vi "Acquisition-ACQUIRE case.vi"(1 "Message Queues":T1, 5 "Logging queue in":T3, 9 "Acquired z-plane index":i32) -> (4 "Imaging Protocol":T2=enum."Live Imaging", 6 "VI Exec time":u32, 10 "Index of next Z-plane to acquire":i32, 15 "Error Out":errorcluster)   [LabVIEW 2020]
doc: "Perform the acquisition. Replace the contents of this diagram with calls to acquisition hardware."
uses:
  Typedefs/Data queue ref.ctl
  Typedefs/Logging queue element.ctl
  Typedefs/Imaging Protocols enum.ctl
  Typedefs/Frame Size.ctl
  Typedefs/Acquired points count.ctl
  User Interface/Queue/Message Queue/Typedefs/All Message Queues.ctl
  User Interface/Queue/Message Queue/Typedefs/Message Cluster.ctl
  Typedefs/HW config states enum.ctl
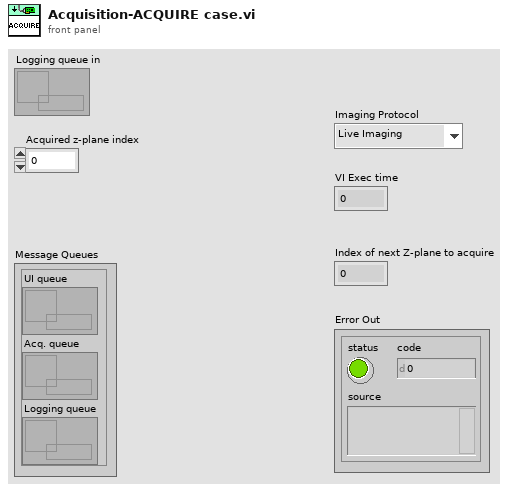
[diagram p1: front panel]
types:
  T1 = typedef "All Message Queues.ctl" = cluster{"UI queue":refnum<queue>, "Acq. queue":refnum<queue>, "Logging queue":refnum<queue>}
  T2 = typedef "Imaging Protocols enum.ctl" = enum16{"AOL Z-Stack", "Motor Z Stack", "Functional Acquisition", "Single Plane Acquisition", "Volume Acquisition", "Live Imaging", "Live Plane Imaging", "Live Volume Imaging"}
  T3 = typedef "Data queue ref.ctl" = refnum<queue>
  T4 = typedef "HW config states enum.ctl" = enum16{"Load from file", "Save to file", "Save backup", "Write all", "Read all", "Write XY stage settings", "Write DAQ FPGA settings", "Write Control FPGA settings", "Write Phys Channels", "Write System Config", "Write HW Config", "Save System Config", "Save HW Config", "Clear", "Compare from file"}
  T5 = typedef "AOL_Globals.ctl" = cluster{"Imaging Protocol":T2, "Number of POI":u16, "Number of Miniscans":u16, "Number of Trials":u16, "Number of Cycles ":u64, "# Averaged Frames":u16, "Laser power (%)":u8, "Pockels (V)":dbl, "Acquisition Length (sec)":dbl, "Fill time (us)":dbl, "POI Dwell time (us)":dbl, "Miniscan Dwell time per pixel (us)":dbl, "PMT 1":dbl, "PMT 2":dbl, "Back Apperture (mA)":dbl, "Frame Size":T6, "Center Frequency":dbl, "Field of View (norm)":dbl, "DwellTime (us)":dbl, "Wavelength (nm)":dbl, "Zoom":dbl, "AOL Z":dbl, "AOL Mode":T7, "GridXY":dbl, "GridZ":dbl, "TriggerPeriod (sec)":dbl, "Number of Pixels in Miniscan":u16, "Experiment folder path":path, "X centre":dbl, "Y centre":dbl, "Angle (degrees)":dbl, "Plane Mode":T8, "Threshold":u16[], "Regenerate Chirps":bool, "Rectangle ROI length (pixels)":u16, "Rectangle ROI height (pixels)":u16, "AOD fill":u16, "StartupDelay":i32, "Samples Wait after Trigger":u16, "Slip Cycle":u32, "Add Cycle":bool, "Functional Mode":T9, "Z Start":dbl, "Z Stop":dbl, "# Planes":i32, "Total Pixels":i32, "Variable Miniscan Pixels":u16[], "Use Variable Length":bool, "Use Variable Resolution":bool, "Laser power (%) at Z Start":u8, "Laser power (%) at Z Stop":u8, "Ref Z Step":i8, "Ref Dwell Time (us)":dbl, "Field of View (um)":dbl}
  T6 = typedef "Frame Size.ctl" = u16
  T7 = typedef "AOL modes.ctl" = enum16{"Raster", "Structural", "Pointing", "Mini Scan", "Alignment"}
  T8 = typedef "Plane Mode.ctl" = u16
  T9 = typedef "Functional Mode.ctl" = enum16{"Point", "Line", "Patch", "Plane", "Volume"}
  T10 = typedef "Hardware Configuration settings.ctl" = cluster{"Dev. PC":bool, "Swap XY on stage":bool, "No of AOD":u8, "MC Supported":bool, "Axial MC":bool, "Computer MAC address":string, "Externalise Triggers":bool, "Trigger HW config":T11, "DAQmx Chan":T12, "XY stage available":bool, "XY Stage":T13, "Z stage available":bool, "Z Stage config cluster":T14, "Encoder available":bool, "Encoder":T15, "VidRec available":bool, "Cam VidRec":T16, "Laser Power Control HW config":T17, "Laser 1 available":bool, "Laser 1 config cluster":T18, "Prechirper 1 available":bool, "Prechirper 1 config cluster":T19, "Control system.FPGA available?":bool, "Control Sys. HW config":T20, "DAQ FPGA HW Config":T21, "PMT Voltage Range":T25}
  T11 = typedef "Triggers HW config.ctl" = cluster{"Available Device List":i32, "Device Address":string}
  T12 = typedef "DAQmx physical channels cluster.ctl" = cluster{"Pockels AO":tag, "Hard shutter AO":tag, "PMT AOs":tag, "Galvo AOs":tag, "Power meter AI":tag}
  T13 = typedef "XY Stage config cluster.ctl" = cluster{"COM port":refnum<visa-resource-name>, "Baudrate":i32, "Type":string}
  T14 = typedef "Z Stage config cluster.ctl" = cluster{"COM port":refnum<visa-resource-name>, "Baudrate":i32, "Type":string}
  T15 = typedef "Encoder config cluster.ctl" = cluster{"IP address":string, "Port":u16, "Wheel radius (cm)":dbl, "Encoder Trigger":tag}
  T16 = typedef "Cam VidRec HW config setup cluster.ctl" = cluster{"DO flag-Video record":tag, "DO flag-Trial start":tag}
  T17 = typedef "Laser Power Control HW config.ctl" = cluster{"Laser Power Control":string, "Laser Power Modulation Control":enum16{"NI", "FPGA"}}
  T18 = typedef "Laser 1 config cluster.ctl" = cluster{"COM port":refnum<visa-resource-name>, "Baud Rate":i32, "Type":string}
  T19 = typedef "PreChirper 1 config cluster.ctl" = cluster{"Type":string, "Baud Rate":i32, "COM port":refnum<visa-resource-name>}
  T20 = typedef "Control Sys HW config cluster.ctl" = cluster{"Control system.FPGA Type":enum16{"Virtex 5", "Virtex 7"}, "Control system.Network adapter name":string, "Control system.MAC address":string, "Control system.Ethernet Port":u32, "Control system.Ethernet Port Opened":bool}
  T21 = typedef "DAQ FPGA HW config cluster.ctl" = cluster{"FGPA Ref":T22, "Target":T23, "input card type":T24}
  T22 = typedef "FPGA Ref.ctl" = refnum<k20>
  T23 = typedef "nirio_resource_hc.ctl" = tag
  T24 = typedef "FPGA input type AC-DC.ctl" = enum16{"AC Card", "DC Card"}
  T25 = typedef "PMT Voltage Range.ctl" = cluster{"PMT Voltage Lower Limit":dbl, "PMT Voltage Upper Limit":dbl}
  T26 = typedef "Logging queue element.ctl" = cluster{"Imaging Protocol":T2, "Number of Trials":u16, "Frame Size":T6, "# Averaged frames":u16, "Dwell time (us)":dbl, "Index of Z-plane":i32, "Timelapse?":bool, "Logging process is active":bool, "Speed logging enabled":bool, "tdms file ref":refnum<k34>, "path":path, "Trial Number":i32, "Expected # points acquired":bool, "Manually stopped":bool, "Last trial":bool, "Ch0 data":u32[], "Ch1 data":u32[], "Ref Data":u32[], "Ref Frame Time":u64[], "Image Time":u64[], "Continuous Time":u64[], "Ref X Length":u16, "Ref Y Length":u16, "# Ref Averaged frames":u16, "Ref Dwell time (us)":dbl, "Points acquired":T27, "HW Timings File":refnum<file>}
  T27 = typedef "Acquired points count.ctl" = cluster{"Ch0 last trial":u64, "Ch1 last trial":u64, "All trials":u64}
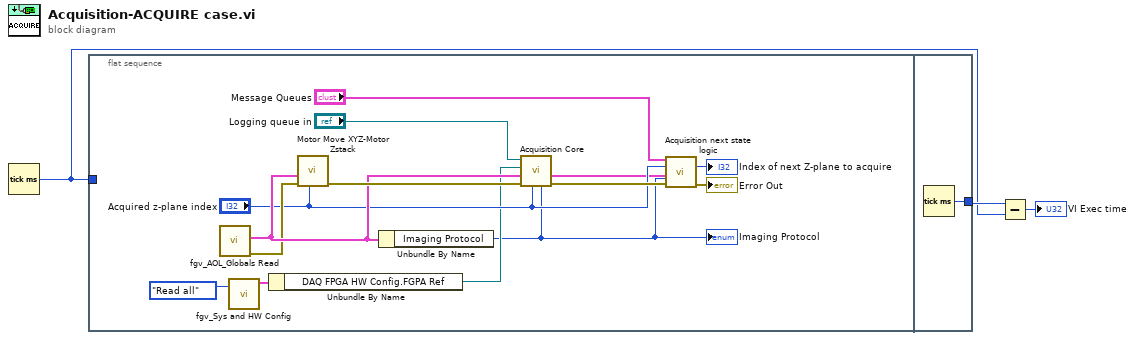
[diagram p0: block diagram]
diagram:
  n1 = Tick Count (ms)() -> (millisecond timer value=w1:u32)
  n2 = flat-sequence {
    tunnel: w1 -> [_]
    tunnel: [w18] -> w3
    frame #0 {
      n3 = call "fgv_AOL_Globals Read.vi"() -> ("error out"=w12:errorcluster, "AOL_Globals"=w16:T5)  [unwired: 9 in, 1 out]
      n4 = call "fgv_Sys and HW Config.vi"("Function"=HW_config_states_enum."Read all") -> ("Hardware Configuration OUT"=w6:T10)  [unwired: 8 in, 2 out]
      n5 = Unbundle By Name(w6) -> ("DAQ FPGA HW Config.FGPA Ref"=w5:T22)
      n6 = call "Motor Move XYZ-Motor Zstack.vi"("Zplane in"="Acquired z-plane index", "error in (no error)"=w12, "AOL_Globals"=w16) -> ("error out"=w17:errorcluster)  [unwired: 8 in]
      n7 = Unbundle By Name(w16) -> ("Imaging Protocol"=w4:T2)
      "Imaging Protocol" <- w4
      n8 = call "Acquisition Core.vi"("Imaging Protocol"=w4, "Acquired z-plane index"="Acquired z-plane index", "error in"=w17, "AOL_Globals"=w16, "FPGA VI Ref"=w5, "Logging queue in"="Logging queue in") -> ("error out"=w15:errorcluster, "Logging queue element"=w8:T26)  [unwired: 4 in]
      n9 = call "Acquisition next state logic.vi"("Message Queues"="Message Queues", "Acquired z-plane index"="Acquired z-plane index", "Logging queue element"=w8, "Imaging Protocol"=w4, "error in"=w15) -> ("Index of next Z-plane to acquire"=→"Index of next Z-plane to acquire":i32, "error out"=→"Error Out":errorcluster)  [unwired: 9 in]
    }
    frame #1 {
      n10 = Tick Count (ms)() -> (millisecond timer value=w18:u32)
    }
  }
  n11 = Subtract(x=w3, y=w1) -> (x-y=→"VI Exec time":u32)
